vi "StopMotor.vi"(8 "error in (no error)":errorcluster) -> (0 "error out":errorcluster, 3 "Stopped":bool)   [LabVIEW 2015]
uses:
  Controls/Mark10 Comm states.ctl
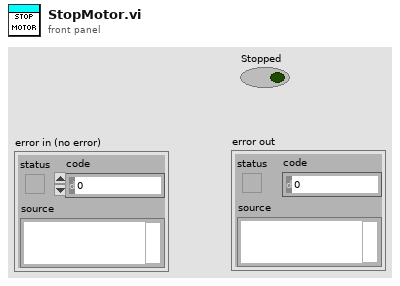
[diagram p1: front panel]
types:
  T1 = typedef "Mark10 Comm states.ctl" = enum16{"Open Session", "Get Reference", "Write Data", "Read Data", "Close Session"}
  T2 = cluster{"MovingUp":bool, "MovingDown":bool, "Stopped":bool, "CycleMode":bool, "LimitMode":bool, "ManualMode":bool, "UpperLimit":bool, "LowerLimit":bool}
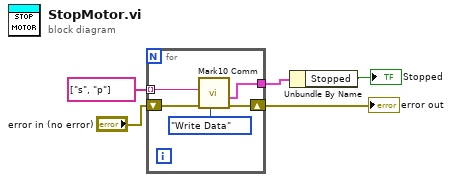
[diagram p0: block diagram]
diagram:
  n1 = for {
    tunnel: string[] ["s", "p"] -> [w9] mode=indexing
    shift-right: [w8] -> w3
    shift-left: "error in (no error)" -> [w7]
    tunnel: [w6] -> w4
    n2 = call "Mark10 Comm.vi"("Action"=Mark10_Comm_states."Write Data", "error in (no error)"=w7, "Write"=w9) -> ("error out"=w8:errorcluster, "Flags"=w6:T2)  [unwired: 2 in, 5 out]
  }
  "error out" <- w3
  n3 = Unbundle By Name(w4) -> ("Stopped"=→"Stopped":bool)
